vi "dispose client connector.vi"(8 "error in":errorcluster, 11 "client connector in":refnum<class "client connector.lvclass">) -> (0 "error out":errorcluster)   [LabVIEW 2016, in "client connector.lvclass"]
uses:
  client connector.lvclass
  C:/Users/IEUser/Desktop/libasynclvtls/tls classes/connection creator/connection creator.lvclass
  dllwrapper/library path.vi
  <vilib>/Utility/error.llb/Error Cluster From Error Code.vi
  dllwrapper/async tls dl.lvlib
  connection creator.lvclass
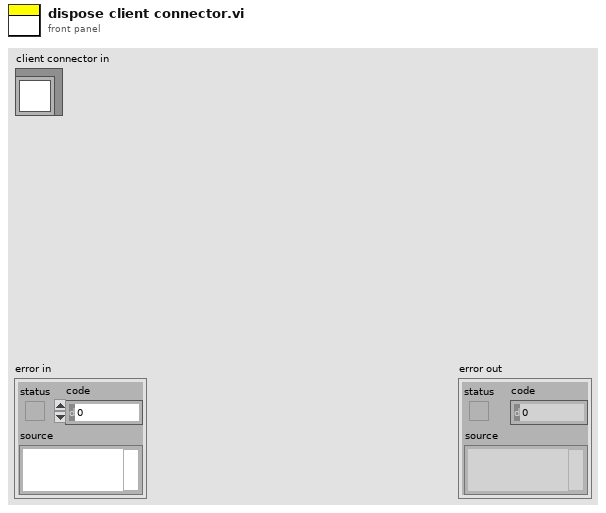
[diagram p1: front panel]
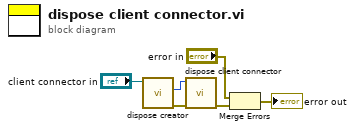
[diagram p0: block diagram]
diagram:
  n1 = call "dispose creator.vi"("connection creator in"="client connector in") -> ("error out"=w3:errorcluster, "pointer"=w2:u64)  [unwired: 9 in]
  n2 = call "dispose client connector.vi"("error in"=w3, "client"=w2) -> ("error out"=w4:errorcluster)  [unwired: 9 in]
  n3 = Merge Errors("error in", w4) -> (→"error out":errorcluster)
